vi "Algorithm_1_sort.vi"() -> ()   [LabVIEW 2020]
panel:
  out "Sorted index":u8[](array[numeric])
  out "Array":i32[](array[numeric])
  out "Output Valid 2":bool
  out "Sorted array 3":u8[](array[numeric])
  in  "Input Array 3":u8[](array[numeric])=[0, 0, 0, 0, 0, 0, 0, 0]
  out "output array":u8[](array[numeric])
  out "Numeric":i32
  out "Sorted array 2":u8[](array[numeric])
  in  "Input Array 2":u8[](array[numeric])=[0, 0, 0, 0, 0, 0, 0, 0]
  out "Sorted array":u8[](array[numeric])
  out "Output Valid":bool
  in  "Input Array":u8[](array[numeric])=[0, 0, 0, 0, 0, 0, 0, 0]
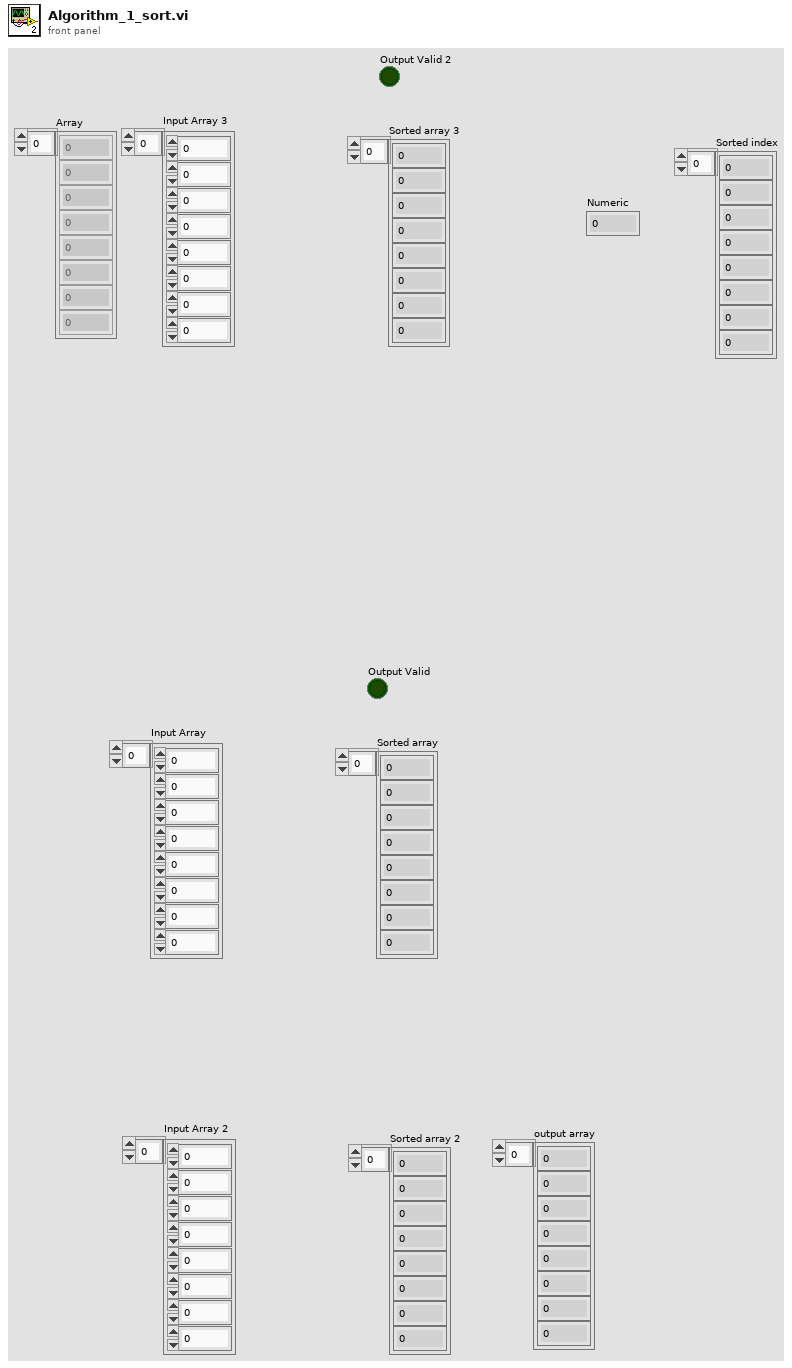
[diagram p1: front panel]
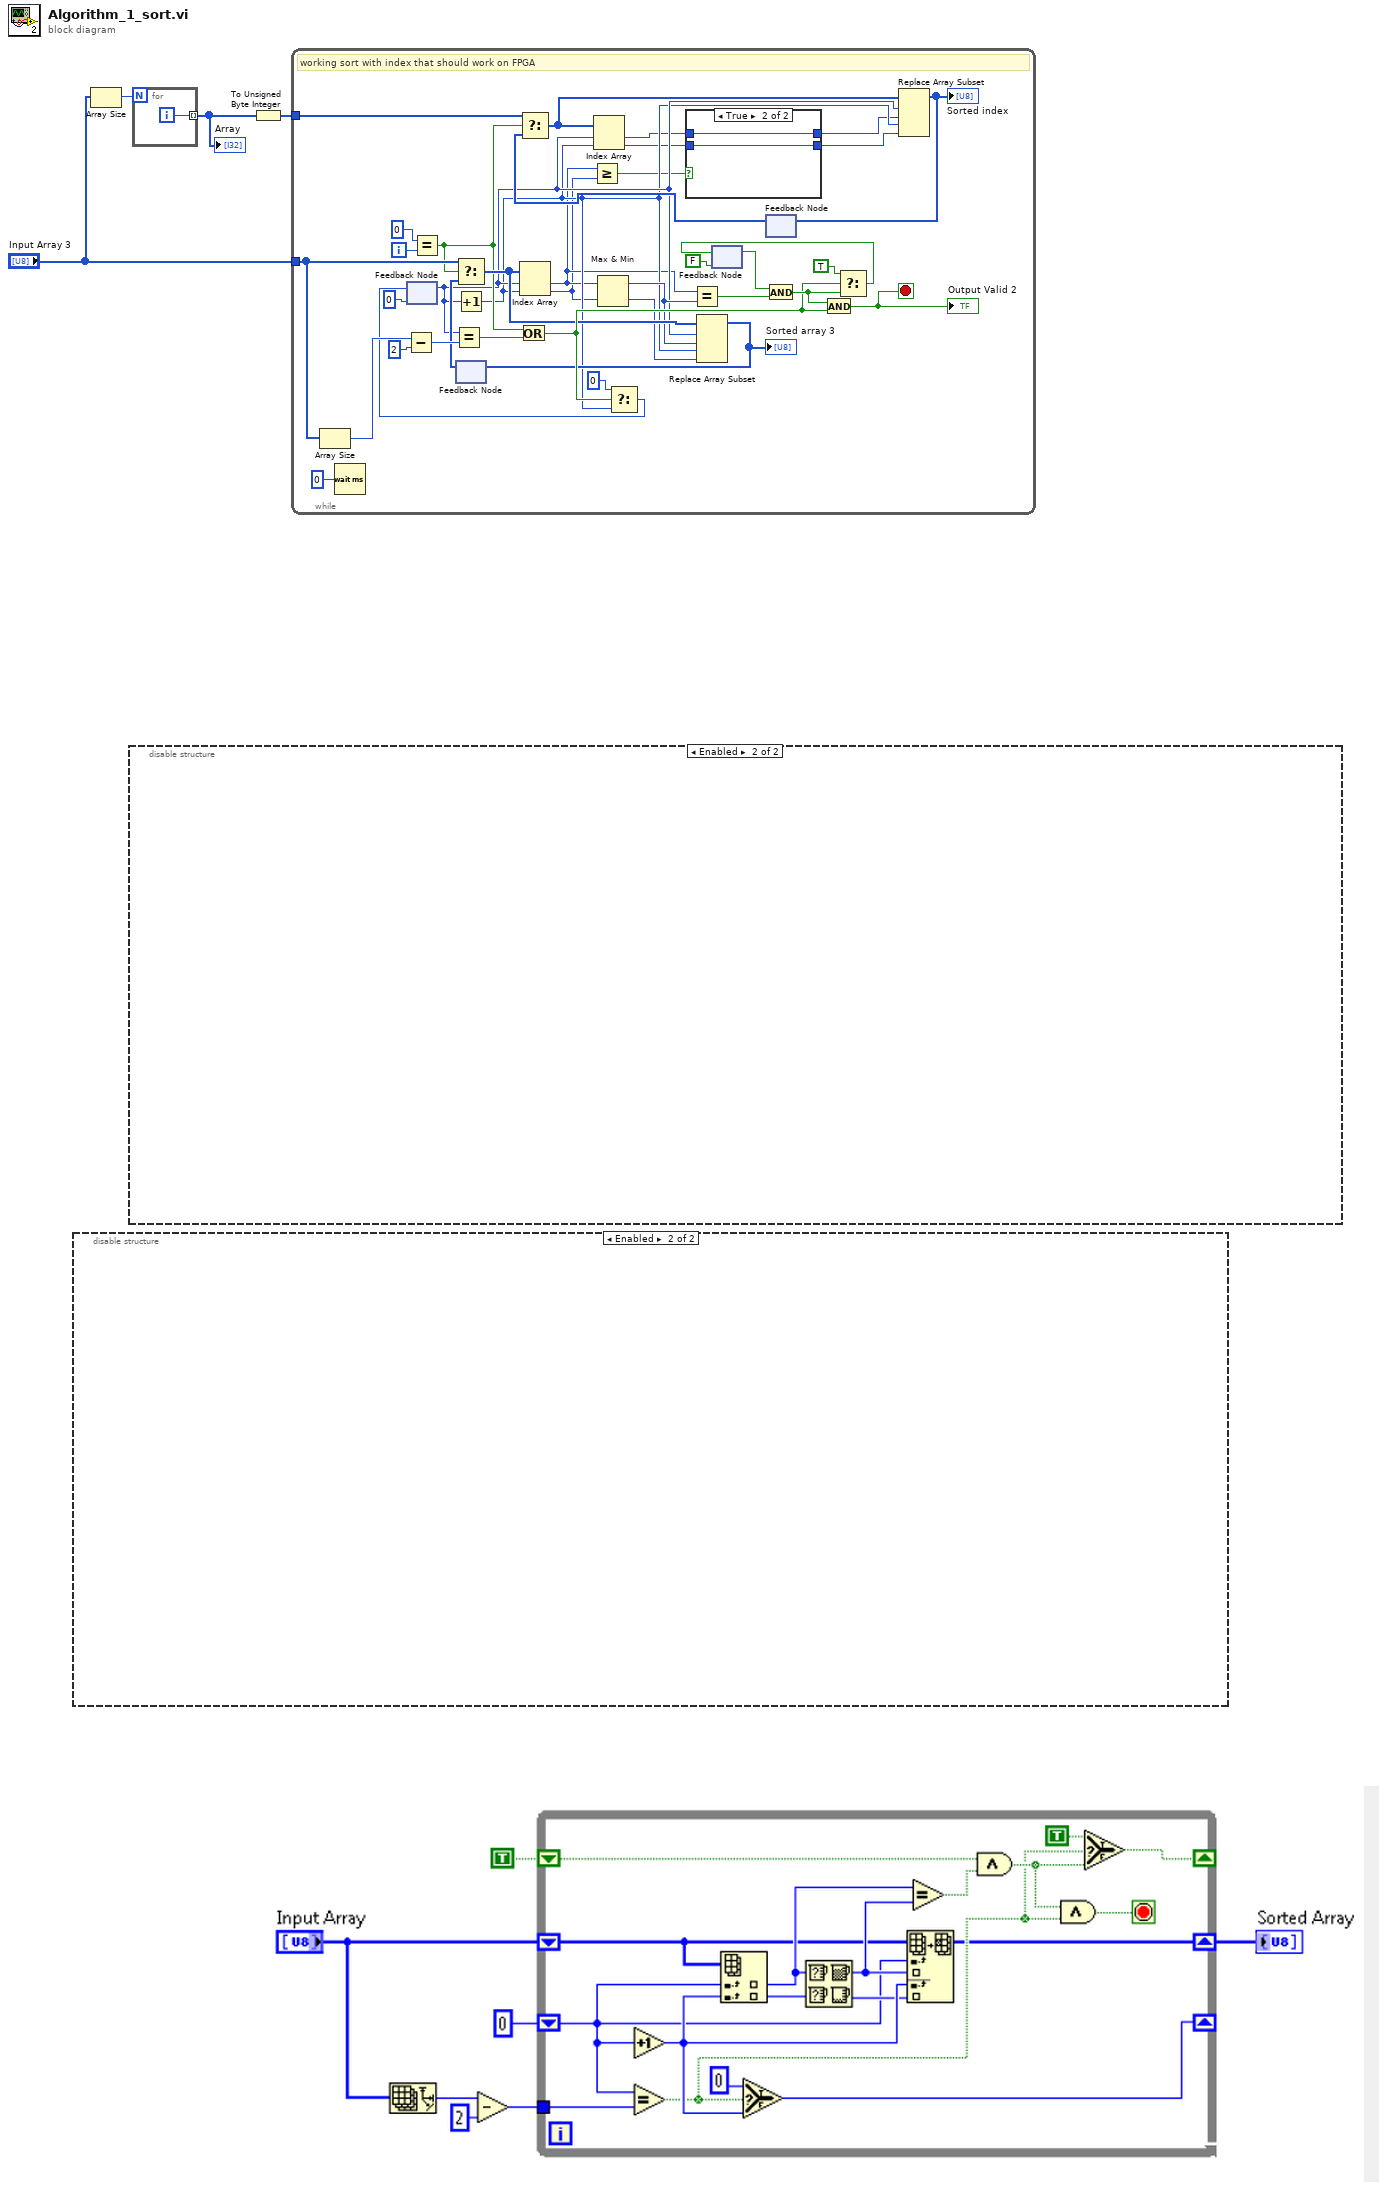
[diagram p0: block diagram]
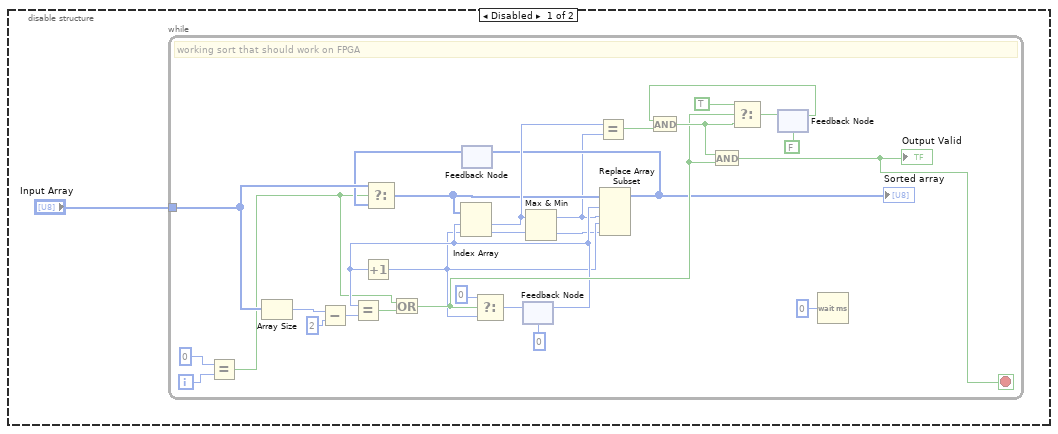
[diagram p3: hidden frame]
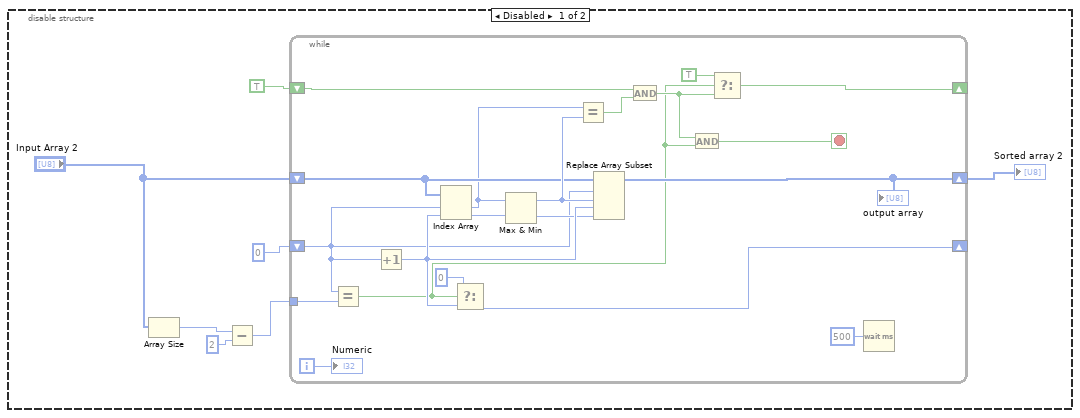
[diagram p4: hidden frame]
diagram:
  n1 = disable-structure shown="Enabled" {
    frame Disabled {
      n2 = Array Size(array="Input Array 2") -> (size(s)=w11:i32)
      n3 = Subtract(x=w11, y=2) -> (x-y=w9:i32)
      n4 = while {
        tunnel: w9 -> [w31]
        shift-right: [w27] -> w7
        shift-left: "Input Array 2" -> [w19]
        shift-right: [w22] -> _
        shift-left: TRUE ("t") -> [w21]
        shift-right: [w16] -> _
        shift-left: 0 ("y") -> [w15]
        i -> [w14]
        stop <- w20 stop-if-true
        n5 = Equal?(x=w15, y=w31) -> (x = y?=w13:bool)
        n6 = Increment(x=w15) -> (x+1=w25:i32)
        n7 = Index Array(array=w19, index #1=w15, index #2=w25) -> (element #1=w17:u8, element #2=w18:u8)
        n8 = Select(t=0 ("y"), s=w13, f=w25) -> (s? t:f=w16:i32)
        n9 = Max & Min(x=w17, y=w18) -> (max(x,y)=w26:u8, min(x,y)=w24:u8)
        n10 = Equal?(x=w17, y=w26) -> (x = y?=w30:bool)
        n11 = Replace Array Subset(array=w19, new element #1=w26, index #1=w15, new element #2=w24, index #2=w25) -> (w27:u8[])
        "output array" <- w27
        n12 = And(x=w21, y=w30) -> (x .and. y?=w29:bool)
        n13 = And(x=w29, y=w13) -> (x .and. y?=w20:bool)
        n14 = Select(t=TRUE, s=w13, f=w29) -> (s? t:f=w22:bool)
        n15 = Wait (ms)(milliseconds to wait=u32 500) -> ()  [unwired: 1 out]
        "Numeric" <- w14
      }
      "Sorted array 2" <- w7
    }
    frame Enabled {
    }
  }
  n16 = Array Size(array="Input Array 3") -> (size(s)=w3:i32)
  n17 = disable-structure shown="Enabled" {
    frame Disabled {
      n18 = while {
        tunnel: "Input Array" -> [w58]
        i -> [w35]
        stop <- w36 stop-if-true
        # "working sort that should work on FPGA"
        n19 = Equal?(x=0, y=w35) -> (x = y?=w33:bool)
        n20 = Array Size(array=w58) -> (size(s)=w61:i32)
        n21 = Subtract(x=w61, y=2) -> (x-y=w59:i32)
        n22 = feedback #1() -> (w49:u8[])  [unwired: 1 in]
        n23 = Select(t=w58, s=w33, f=w49) -> (s? t:f=w43:u8[])
        n24 = feedback #2(0 ("y")) -> (w41:i32)
        n25 = Equal?(x=w41, y=w59) -> (x = y?=w44:bool)
        n26 = Increment(x=w41) -> (x+1=w39:i32)
        n27 = Or(x=w33, y=w44) -> (x .or. y?=w47:bool)
        n28 = Index Array(array=w43, index #1=w41, index #2=w39) -> (element #1=w56:u8, element #2=w57:u8)
        n29 = Select(t=0 ("y"), s=w47, f=w39) -> (s? t:f=w45:i32)
        n30 = feedback-in #2(w45) -> ()
        n31 = Max & Min(x=w56, y=w57) -> (max(x,y)=w40:u8, min(x,y)=w38:u8)
        n32 = Equal?(x=w56, y=w40) -> (x = y?=w55:bool)
        n33 = Replace Array Subset(array=w43, new element #1=w40, index #1=w41, new element #2=w38, index #2=w39) -> (w42:u8[])
        "Sorted array" <- w42
        n34 = feedback-in #1(w42) -> ()
        n35 = feedback #3(FALSE ("t")) -> (w52:bool)
        n36 = And(x=w52, y=w55) -> (x .and. y?=w50:bool)
        n37 = And(x=w50, y=w47) -> (x .and. y?=w36:bool)
        "Output Valid" <- w36
        n38 = Select(t=TRUE, s=w47, f=w50) -> (s? t:f=w53:bool)
        n39 = feedback-in #3(w53) -> ()
        n40 = Wait (ms)(milliseconds to wait=u32 0) -> ()  [unwired: 1 out]
      }
    }
    frame Enabled {
    }
  }
  n41 = for {
    N: w3 -> [_]
    tunnel: [w62] -> w2 mode=indexing
    i -> [w62]
  }
  "Array" <- w2
  n42 = To Unsigned Byte Integer(number=w2) -> (unsigned 8bit integer=w1:u8[])
  n43 = while {
    tunnel: "Input Array 3" -> [w97]
    tunnel: w1 -> [w74]
    i -> [w78]
    stop <- w79 stop-if-true
    # "working sort with index that should work on FPGA"
    n44 = Array Size(array=w97) -> (size(s)=w100:i32)
    n45 = Wait (ms)(milliseconds to wait=u32 0) -> ()  [unwired: 1 out]
    n46 = Subtract(x=w100, y=2) -> (x-y=w98:i32)
    n47 = feedback #4(0 ("y")) -> (w72:i32)
    n48 = Equal?(x=0, y=w78) -> (x = y?=w73:bool)
    n49 = Equal?(x=w72, y=w98) -> (x = y?=w85:bool)
    n50 = Increment(x=w72) -> (x+1=w71:i32)
    n51 = feedback #5() -> (w90:u8[])  [unwired: 1 in]
    n52 = Select(t=w97, s=w73, f=w90) -> (s? t:f=w84:u8[])
    n53 = Or(x=w73, y=w85) -> (x .or. y?=w88:bool)
    n54 = Index Array(array=w84, index #1=w72, index #2=w71) -> (element #1=w65:u8, element #2=w64:u8)
    n55 = Greater Or Equal?(x=w65, y=w64) -> (x >= y?=w63:bool)
    n56 = Max & Min(x=w65, y=w64) -> (max(x,y)=w82:u8, min(x,y)=w81:u8)
    n57 = Select(t=0 ("y"), s=w88, f=w71) -> (s? t:f=w86:i32)
    n58 = feedback-in #4(w86) -> ()
    n59 = Equal?(x=w65, y=w82) -> (x = y?=w96:bool)
    n60 = Replace Array Subset(array=w84, new element #1=w82, index #1=w72, new element #2=w81, index #2=w71) -> (w83:u8[])
    "Sorted array 3" <- w83
    n61 = feedback-in #5(w83) -> ()
    n62 = feedback #6(FALSE ("t")) -> (w93:bool)
    n63 = feedback #7() -> (w76:u8[])  [unwired: 1 in]
    n64 = Select(t=w74, s=w73, f=w76) -> (s? t:f=w75:u8[])
    n65 = Index Array(array=w75, index #1=w72, index #2=w71) -> (element #1=w69:u8, element #2=w66:u8)
    n66 = case shown="True" w63 {
      tunnel: w69 -> [w102 w104]
      tunnel: [w101 w104] -> w68
      tunnel: [w102 w103] -> w67
      tunnel: w66 -> [w101 w103]
      frame False {
      }
      frame True {
      }
    }
    n67 = And(x=w93, y=w96) -> (x .and. y?=w91:bool)
    n68 = And(x=w91, y=w88) -> (x .and. y?=w79:bool)
    "Output Valid 2" <- w79
    n69 = Select(t=TRUE, s=w88, f=w91) -> (s? t:f=w94:bool)
    n70 = feedback-in #6(w94) -> ()
    n71 = Replace Array Subset(array=w75, new element #1=w68, index #1=w72, new element #2=w67, index #2=w71) -> (w70:u8[])
    "Sorted index" <- w70
    n72 = feedback-in #7(w70) -> ()
  }
